vi "Update Configuration.vi"(6 "timeout (ms)":i32=5000, 8 "error in":errorcluster, 10 "JSON Configuration":string, 11 "gRPC ID":T1) -> (0 "error out":errorcluster, 3 "gRPC ID out":T1)   [LabVIEW 2021, in "CoreGrpcClientWrapper.lvlib"]
uses:
  <vilib>/gRPC/LabVIEW gRPC Library/Shared/grpcId.ctl
  CoreGrpcClientWrapper.lvlib
  CIF_Plugin_Core_client/CIF_Plugin_Core_client.lvlib
  CIF_Plugin_Core_client/RPC Messages/cif_plugincore_Configuration.ctl
  <vilib>/gRPC/LabVIEW gRPC Library/grpc-lvsupport-release.lvlib
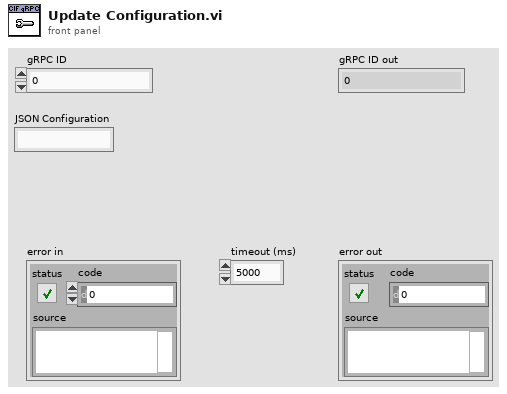
[diagram p1: front panel]
types:
  T1 = typedef "grpc-lvsupport-release.lvlib/grpcId.ctl" = u64
  T2 = typedef "CIF_Plugin_Core_client.lvlib/cif_plugincore_Configuration.ctl" = cluster{"json_config":string}
  T3 = typedef "CIF_Plugin_Core_client.lvlib/cif_plugincore_Status.ctl" = cluster{"code":i32, "message":string}
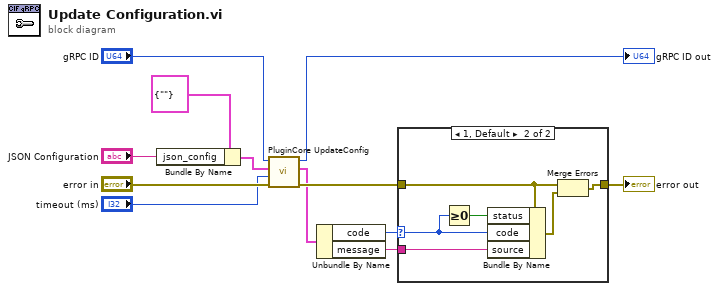
[diagram p0: block diagram]
diagram:
  n1 = Bundle By Name(cluster=T2 {"json_config"=""} ("Request Data"), "json_config"="JSON Configuration") -> (w1:T2)
  n2 = call "PluginCore UpdateConfig.vi"("error in"="error in", "timeout (ms)"="timeout (ms)", "Request Data"=w1, "gRPC ID"="gRPC ID") -> ("error out"=w7:errorcluster, "Response Data"=w4:T3, "gRPC ID out"=→"gRPC ID out":T1)  [unwired: 5 in]
  n3 = Unbundle By Name(w4) -> ("code"=w5:i32, "message"=w8:string)
  n4 = case shown="1, Default" w5 {
    selector: w5 -> [_ w14]
    tunnel: w8 -> [_ w18]
    tunnel: w7 -> [w13 w17]
    tunnel: [w13 w15] -> w6
    frame 0 {
    }
    frame 1, Default {
      n5 = Greater Or Equal To 0?(x=w14) -> (x >= 0?=w19:bool)
      n6 = Bundle By Name(cluster=w17, "status"=w19, "code"=w14, "source"=w18) -> (w16:errorcluster)
      n7 = Merge Errors(w17, w16) -> (w15:errorcluster)
    }
  }
  "error out" <- w6
